vi "PositionOffset__slk_mt.vi"(3 "position in":cluster{"X":i32, "Y":i32}, 4 "vertical arrangement":T1(ring)) -> (5 "position out":cluster{"X":i32, "Y":i32})   [LabVIEW 2015, in "Lazyboots Menu Tool.lvlib" / "Label__slk_mt.lvclass"]
doc: "Adds the offset to the position by specified vertical arragement."
uses:
  <vilib>/SLK/Lazyboots Menu Tool/Private/AddLabel/Class/Label/Label__slk_mt.lvclass
panel:
  # "PositionOffset__slk_mt.vi\nAdds the offset to the position by specified vertical arragement.\n\nNOTICE -- YOU MUST LEAVE THIS NOTICE IN PLACE.\n\nCopyright (c) 2011, LIANG LIU Shawn.Liu.cn@gmail.com\nAll rights reserved.\n\nRedistribution and use in source and binary forms, with or without modification, are permitted provided that the following conditions are met:\n-Redistributions of source code must retain the above copyright notice, this list of conditions and the following disclaimer.\n-Redistributions in binary form must reproduce the above copyright notice, this list of conditions and the following disclaimer in the documentation and/or other materials provided with the distribution.\n-Neither the name of the eLp nor the names of its contributors may be used to endorse or promote products derived from this software without specific prior written permission.\n\nTHIS SOFTWARE IS PROVIDED BY THE COPYRIGHT HOLDERS AND CONTRIBUTORS \"AS IS\" AND ANY EXPRESS OR IMPLIED WARRANTIES, INCLUDING, BUT NOT LIMITED TO, THE IMPLIED WARRANTIES OF MERCHANTABILITY AND FITNESS FOR A PARTICULAR PURPOSE ARE DISCLAIMED. IN NO EVENT SHALL THE COPYRIGHT HOLDER OR CONTRIBUTORS BE LIABLE FOR ANY DIRECT, INDIRECT, INCIDENTAL, SPECIAL, EXEMPLARY, OR CONSEQUENTIAL DAMAGES (INCLUDING, BUT NOT LIMITED TO, PROCUREMENT OF SUBSTITUTE GOODS OR SERVICES; LOSS OF USE, DATA, OR PROFITS; OR BUSINESS INTERRUPTION) HOWEVER CAUSED AND ON ANY THEORY OF LIABILITY, WHETHER IN CONTRACT, STRICT LIABILITY, OR TORT (INCLUDING NEGLIGENCE OR OTHERWISE) ARISING IN ANY WAY OUT OF THE USE OF THIS SOFTWARE, EVEN IF ADVISED OF THE POSSIBILITY OF SUCH DAMAGE."
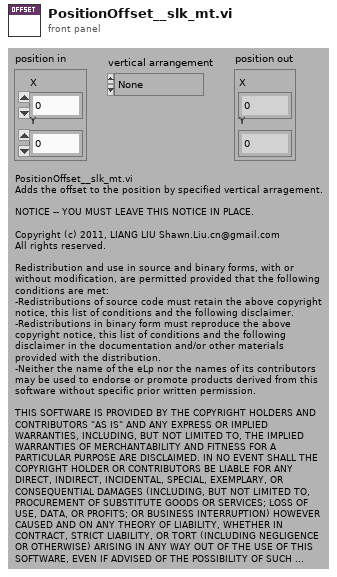
[diagram p1: front panel]
types:
  T1 = enum16{"None", "Stacked", "Clockwise", "Counterclockwise"}
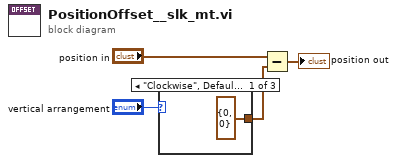
[diagram p0: block diagram]
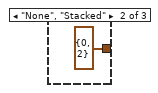
[diagram p2: hidden frame]
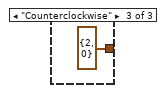
[diagram p3: hidden frame]
diagram:
  n1 = case shown="\"Clockwise\", Default" "vertical arrangement" {
    tunnel: [cluster{"X":i32, "Y":i32} {"X"=0, "Y"=0} ("x") cluster{"X":i32, "Y":i32} {"X"=0, "Y"=2} ("x") cluster{"X":i32, "Y":i32} {"X"=2, "Y"=0} ("x")] -> w2
    frame "Clockwise", Default {
    }
    frame "None", "Stacked" {
    }
    frame "Counterclockwise" {
    }
  }
  n2 = Subtract(x="position in", y=w2) -> (x-y=→"position out":cluster{"X":i32, "Y":i32})
